vi "Comments.Add Experiment Description.vi"(7 "error in (no error)":errorcluster, 10 "AFM Control":refnum<class "AFM Control.lvclass">) -> (0 "error out":errorcluster, 3 "AFM Control out":refnum<class "AFM Control.lvclass">)   [LabVIEW 2016, in "AFM Control.lvclass"]
uses:
  AFM Control.lvclass
  AFM Control.lvclass/AFM Control.ctl
panel:
  out "Experiment Description":string
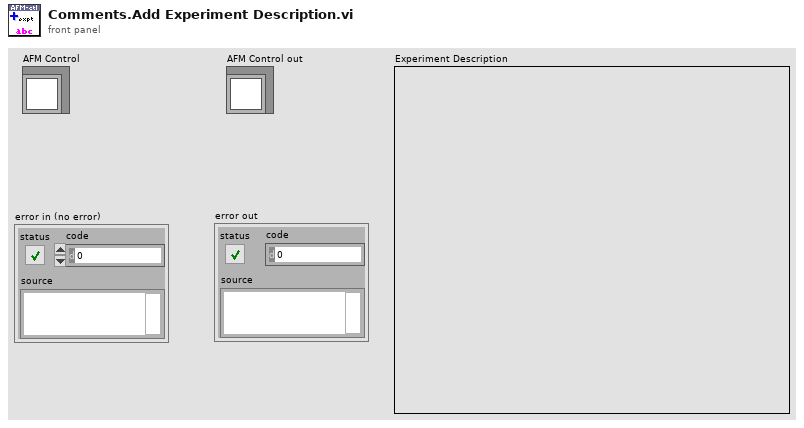
[diagram p1: front panel]
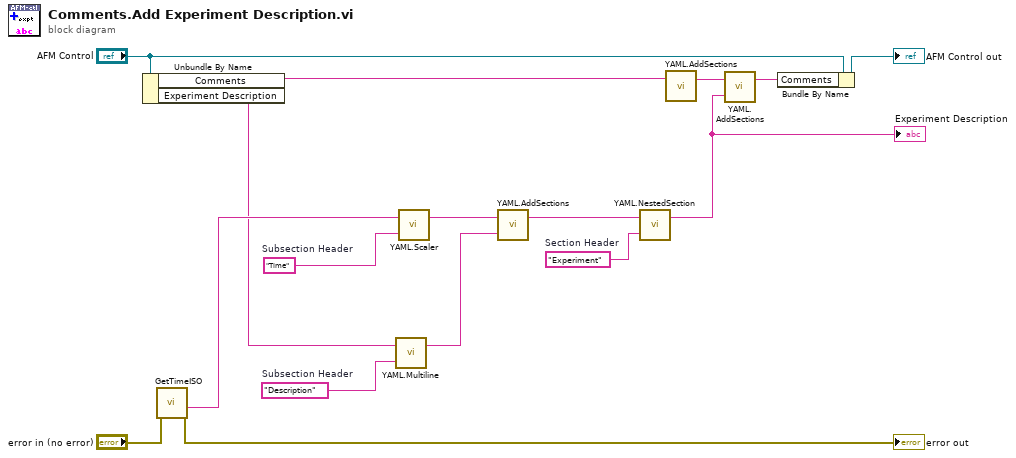
[diagram p0: block diagram]
diagram:
  w6 = "Description"  # Subsection Header
  w7 = "Time"  # Subsection Header
  w5 = "Experiment"  # Section Header
  n1 = Unbundle By Name("AFM Control") -> ("Comments"=w3:string, "Experiment Description"=w1:string)
  n2 = call "GetTimeISO.vi"("error in (no error)"="error in (no error)") -> ("error out"=→"error out":errorcluster, "ISO 8601 date-time string"=w8:string)  [unwired: 8 in, 1 out]
  n3 = call "YAML.Multiline.vi"("Key"=w6, "Multiline"=w1) -> ("Output"=w10:string)  [unwired: 1 in]
  n4 = call "YAML.Scaler.vi"("Key"=w7, "Scaler"=w8) -> ("Output"=w12:string)  [unwired: 1 in]
  n5 = call "YAML.AddSections.vi"("Section 2"=w10, "Section 1"=w12) -> ("Output"=w9:string)  [unwired: 1 in]
  n6 = call "YAML.NestedSection.vi"("Section Key"=w5, "Nested Section"=w9) -> ("String"=w2:string)  [unwired: 1 in]
  "Experiment Description" <- w2
  n7 = call "YAML.AddSections.vi"("Section 1"=w3) -> ("Output"=w4:string)  [unwired: 2 in]
  n8 = call "YAML.AddSections.vi"("Section 2"=w2, "Section 1"=w4) -> ("Output"=w11:string)  [unwired: 1 in]
  n9 = Bundle By Name(cluster="AFM Control", "Comments"=w11) -> (→"AFM Control out":refnum<class "AFM Control.lvclass">)
